vi "欧姆龙PLC通讯Main-TCP.vi"(9 "起始地址16":string="\u0000\u001e\u0000", 10 "数据":dbl[](array[numeric]), 11 "欧姆龙PLC Action":T1) -> (0 "接收数据":string, 1 "读取高度值":i16, 2 "触发信号":bool[](array[boolean]), 3 "PLC连线成功":bool)   [LabVIEW 2014]
uses:
  Controls/MsgAction.ctl
panel:
  out "数组 2":i16[](array[numeric])
  out "数组":i16[](array[numeric])
  out "布尔 2":bool
  out "无符号字节数组 2":u8[](array[numeric])
  out "子字符串 2":string
  out "错误输出 2":errorcluster caption="错误输出"
  in  "接收数据 参考":string="FINS\u0000\u0000\u0000\u001c\u0000\u0000\u0000\u0002\u0000\u0000\u0000\u0000€\u0000\u0002\u0000!\u0000\u0000À\u0000\u0000\u0001\u0002²\u0000\u001e\u0000\u0000\u0001\u0000\u0005"
  out "连接的字符串":string
  out "无符号字节数组":u8[](array[numeric])
  out "子字符串":string
  out "数据长度":string
  out "字符串":string
  out "布尔":bool
  out "错误输出":errorcluster
  out "打开TCP连接成功 2":bool
  out "打开TCP连接成功":bool
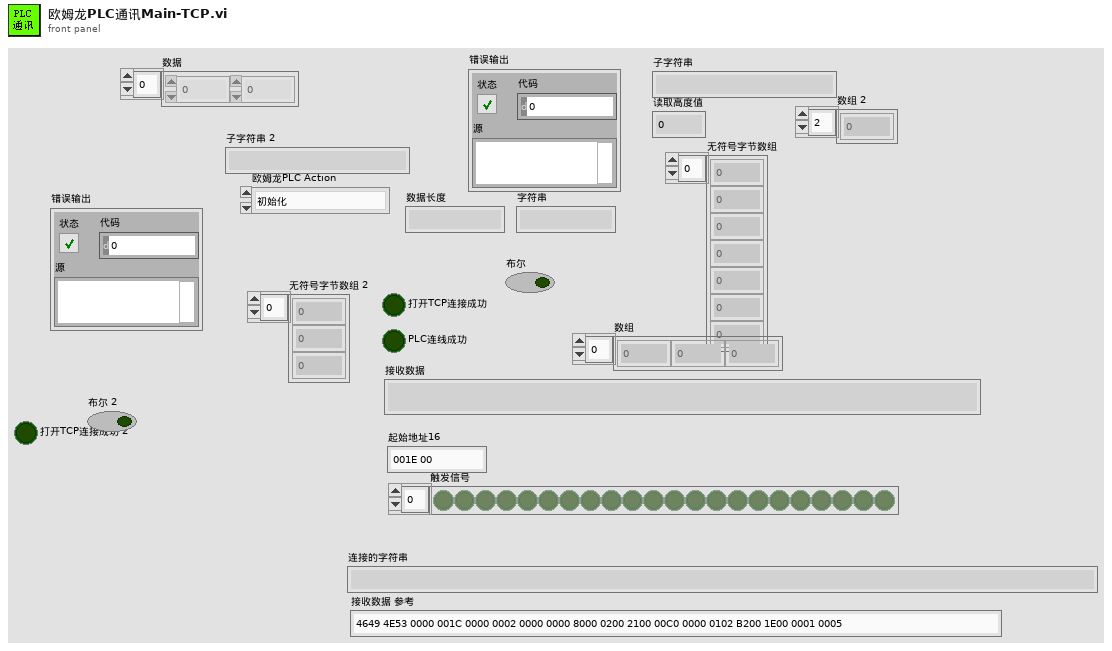
[diagram p1: front panel]
types:
  T1 = typedef "欧姆龙PLC Action.ctl" = enum16{"初始化", "重新初始化", "读触发信息", "读共面度", "写数据", "获取信息"}
  T2 = typedef "MsgAction.ctl" = enum16{"初始化", "添加消息", "区分结果添加消息", "清空消息", "获取消息"}
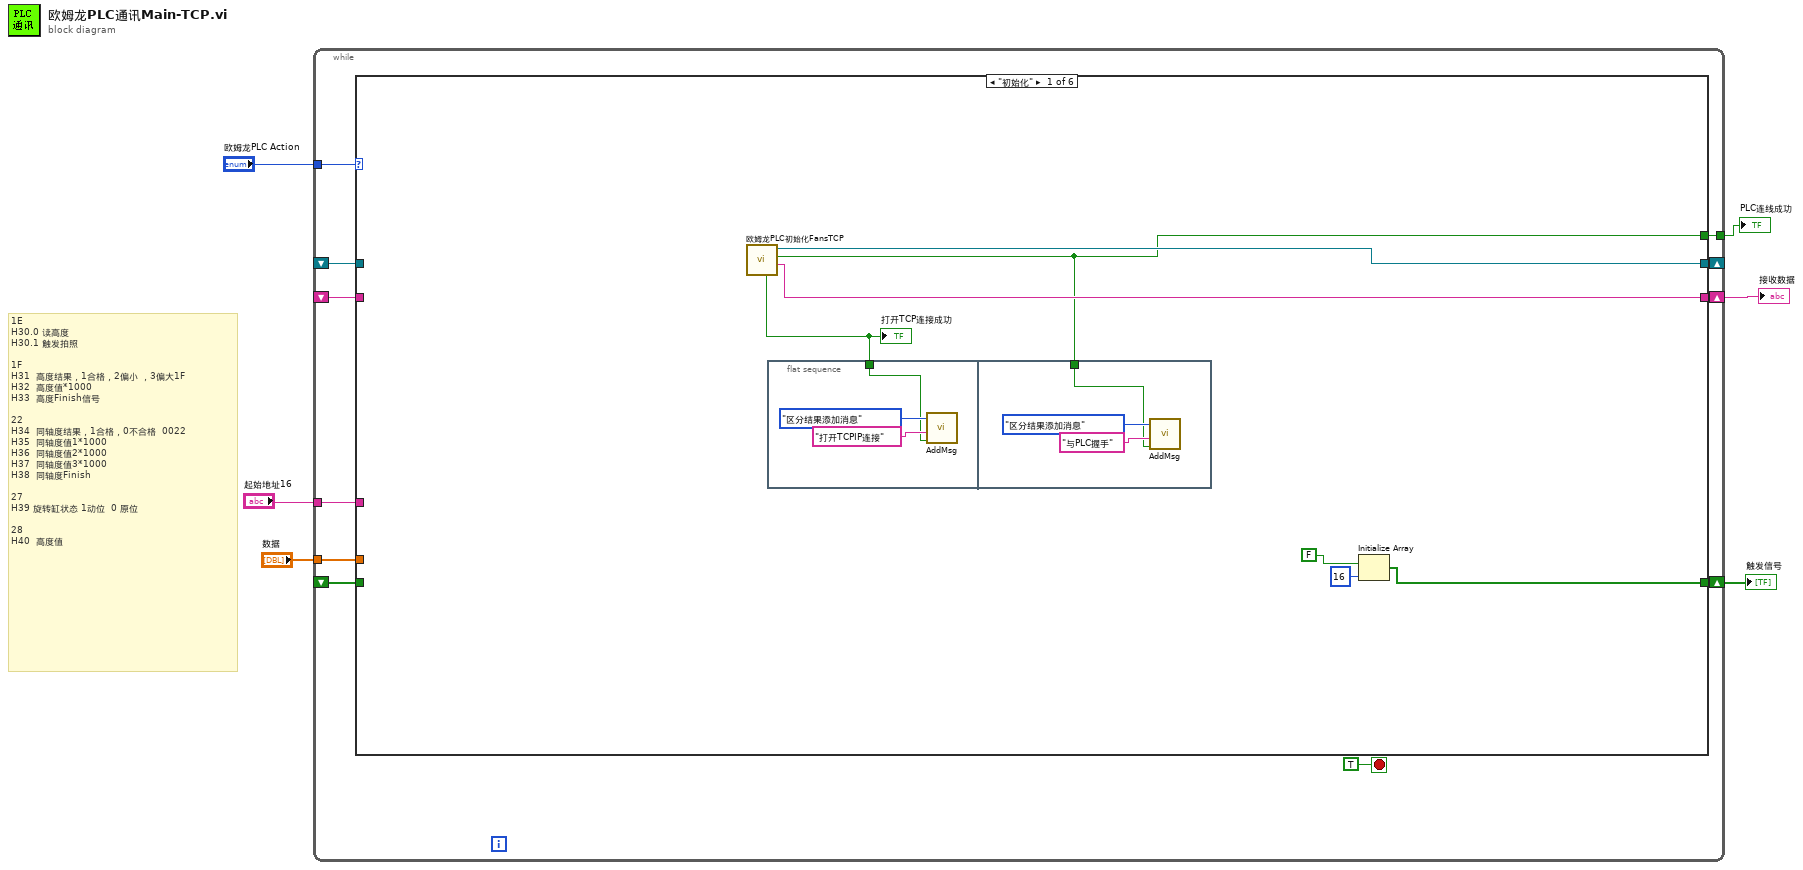
[diagram p0: block diagram]
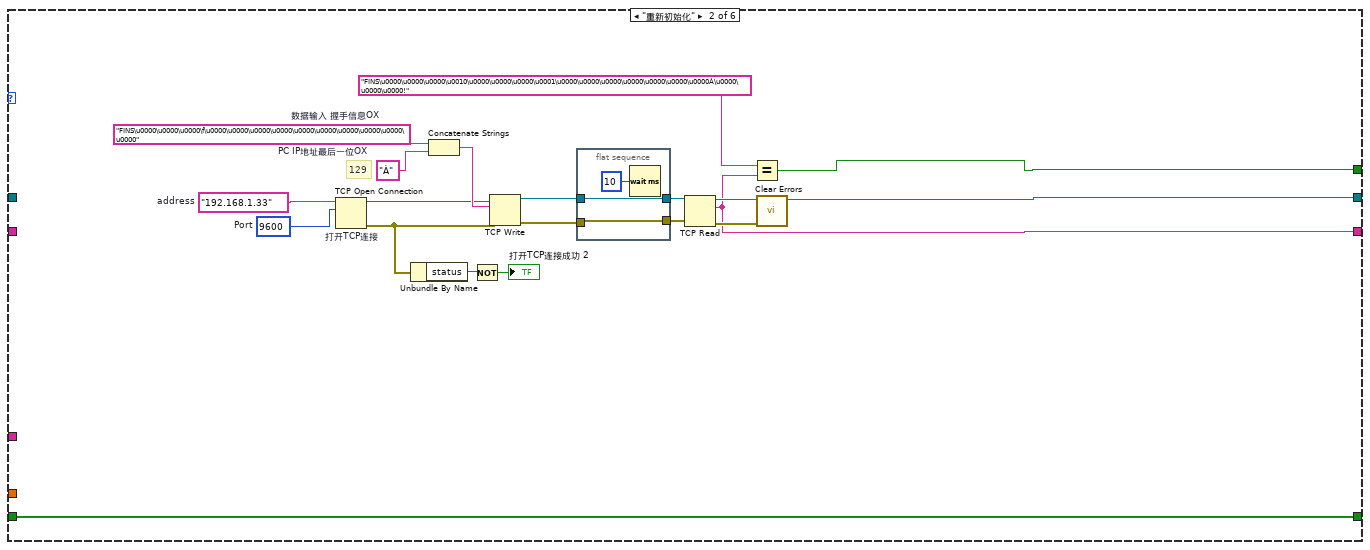
[diagram p2: hidden frame]
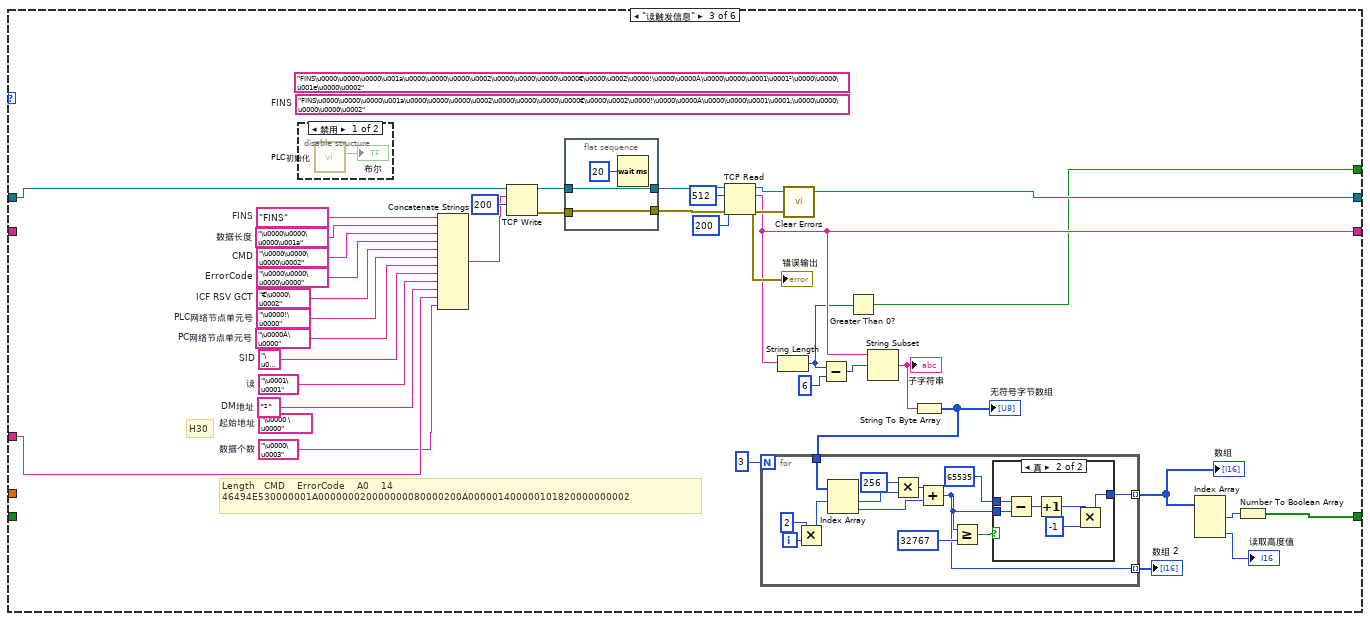
[diagram p3: hidden frame]
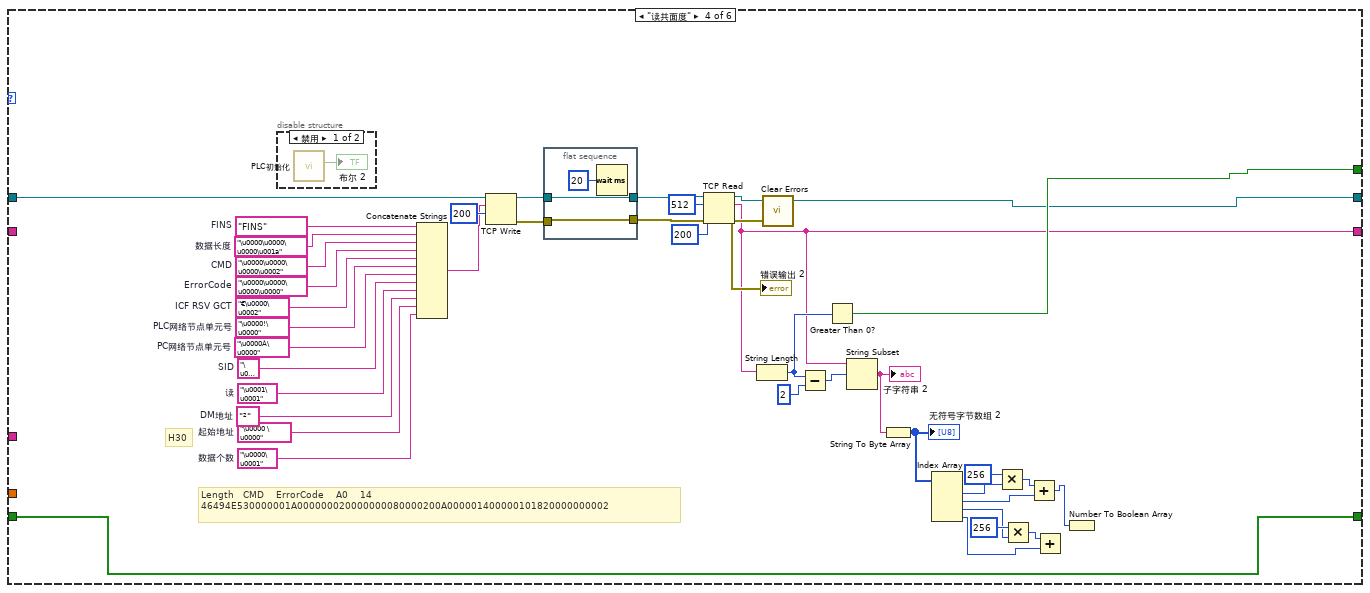
[diagram p6: hidden frame]
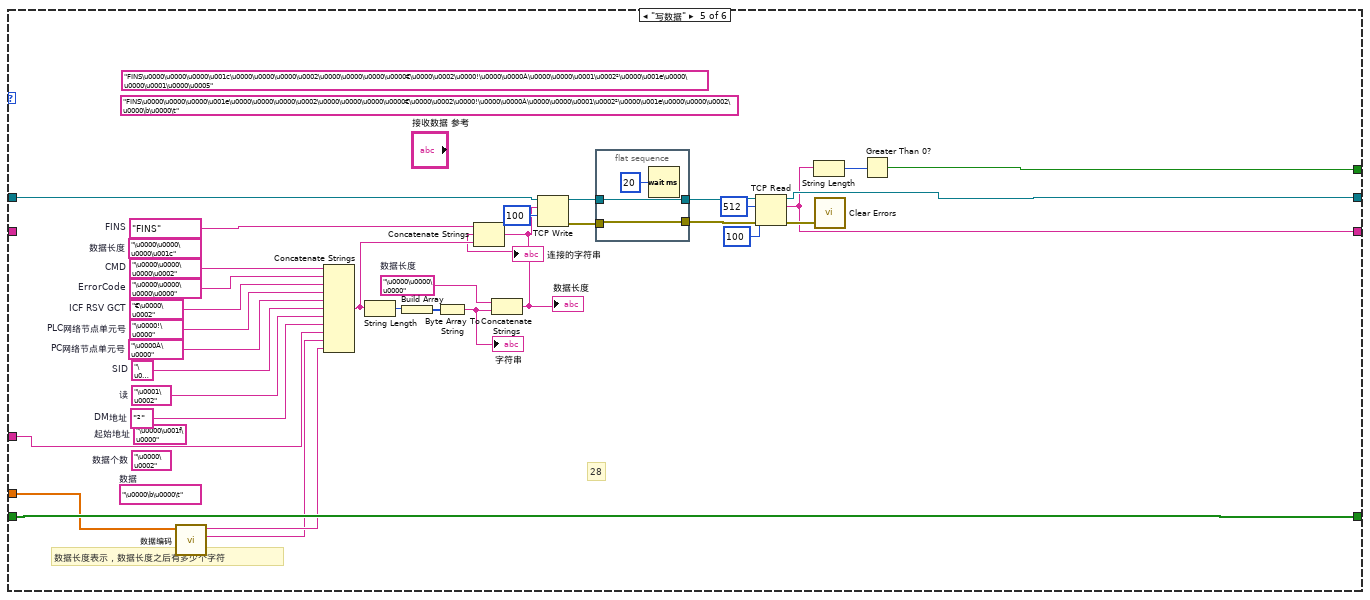
[diagram p8: hidden frame]
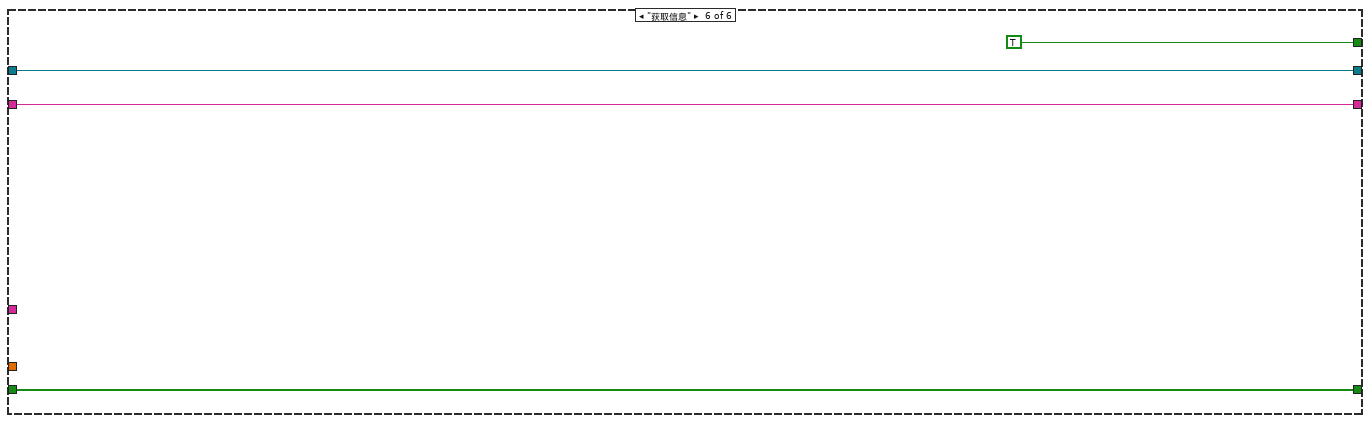
[diagram p9: hidden frame]
diagram:
  # "1E\nH30.0 读高度\nH30.1 触发拍照\n\n1F\nH31  高度结果，1合格，2偏小 ，3偏大1F\nH32  高度值*1000\nH33  高度Finish信号\n\n22\nH34  同轴度结果，1合格，0不合格  0022\nH35  同轴度值1*1000\nH36  同轴度值2*1000\nH37  同轴度值3*1000\nH38  同轴度Finish\n\n27\nH39 旋转缸状态 1动位  0 原位\n\n28\nH40  高度值"
  n1 = while {
    tunnel: "欧姆龙PLC Action" -> [w16]
    shift-right: [w15] -> _
    shift-left: _ -> [w14]
    shift-right: [w13] -> w5
    shift-left: _ -> [w12]
    tunnel: [w11] -> w4
    shift-right: [w10] -> w3
    shift-left: _ -> [w9]
    tunnel: "起始地址16" -> [w8]
    tunnel: "数据" -> [w7]
    stop <- TRUE ("停止") stop-if-true
    n2 = case shown="\"初始化\"" w16 {
      tunnel: [w24 w34 w74 w117 w174 w197] -> w15
      tunnel: w14 -> [_ _ w61 w119 w162 w197]
      tunnel: [w23 w33 w68 w116 w165 w196] -> w13
      tunnel: w12 -> [_ _ _ _ _ w196]
      tunnel: [w18 w32 w62 w118 w163 TRUE ("布尔")] -> w11
      tunnel: [w20 w31 w64 w114 w166 w194] -> w10
      tunnel: w9 -> [_ w31 _ w114 w166 w194]
      tunnel: w8 -> [_ _ w60 _ w161 _]
      tunnel: w7 -> [_ _ _ _ w158 _]
      frame "初始化" {
        n3 = call "欧姆龙PLC初始化FansTCP.vi"() -> ("data out"=w23:string, "布尔"=w18:bool, "TCP网络连接输出"=w24:refnum<k5>, "打开TCP连接成功"=w19:bool)  [unwired: 8 in]
        "打开TCP连接成功" <- w19
        n4 = flat-sequence {
          tunnel: w19 -> [w25]
          tunnel: w18 -> [w28]
          frame #0 {
            n5 = call "AddMsg.vi"("Result"=w25, "添加消息"="打开TCPIP连接" ("消息显示"), "消息Action"=MsgAction."区分结果添加消息") -> ()  [unwired: 1 in, 1 out]
          }
          frame #1 {
            n6 = call "AddMsg.vi"("Result"=w28, "添加消息"="与PLC握手" ("消息显示"), "消息Action"=MsgAction."区分结果添加消息") -> ()  [unwired: 1 in, 1 out]
          }
        }
        n7 = Initialize Array(FALSE, 16 ("维数大小")) -> (w20:bool[])
      }
      frame "重新初始化" {
        w46 = "À"  # PC IP地址最后一位OX
        w47 = "FINS\u0000\u0000\u0000\f\u0000\u0000\u0000\u0000\u0000\u0000\u0000\u0000\u0000\u0000"  # 数据输入 握手信息OX
        w48 = 9600  # Port
        w49 = "192.168.1.33"  # address
        # "129"
        n8 = TCP Open Connection "打开TCP连接"(address=w49, remote port or service name=w48) -> (connection ID=w42:refnum<k5>, error out=w41:errorcluster)  [unwired: 3 in]
        n9 = Unbundle By Name(w41) -> ("status"=w43:bool)
        n10 = Concatenate Strings(w47, w46) -> (w45:string)
        n11 = Not(x=w43) -> (.not. x?=→"打开TCP连接成功 2":bool)
        n12 = TCP Write(connection ID=w42, data in=w45, error in (no error)=w41) -> (connection ID out=w37:refnum<k5>, error out=w39:errorcluster)  [unwired: 1 in, 1 out]
        n13 = flat-sequence {
          tunnel: w39 -> [w52]
          tunnel: [w52] -> w38
          tunnel: w37 -> [w50]
          tunnel: [w50] -> w36
          frame #0 {
            n14 = Wait (ms)(milliseconds to wait=u32 10 ("等待时间（毫秒）")) -> ()  [unwired: 1 out]
          }
        }
        n15 = TCP Read(connection ID=w36, error in (no error)=w38) -> (connection ID out=w34:refnum<k5>, data out=w33:string, error out=w40:errorcluster)  [unwired: 3 in]
        n16 = Equal?(x="FINS\u0000\u0000\u0000\u0010\u0000\u0000\u0000\u0001\u0000\u0000\u0000\u0000\u0000\u0000\u0000À\u0000\u0000\u0000!", y=w33) -> (x = y?=w32:bool)
        n17 = call <vilib>:"Clear Errors.vi"("error in (no error)"=w40) -> ()  [unwired: 5 in, 2 out]
      }
      frame "读触发信息" {
        (unwired) "FINS\u0000\u0000\u0000\u001a\u0000\u0000\u0000\u0002\u0000\u0000\u0000\u0000€\u0000\u0002\u0000!\u0000\u0000À\u0000\u0000\u0001\u0001²\u0000\u0000\u001e\u0000\u0002" ("接收数据 2")
        (unwired) "FINS\u0000\u0000\u0000\u001a\u0000\u0000\u0000\u0002\u0000\u0000\u0000\u0000€\u0000\u0002\u0000!\u0000\u0000À\u0000\u0000\u0001\u0001‚\u0000\u0000\u0000\u0000\u0002"  # FINS
        w59 = "\u0000\u0003"  # 数据个数
        (unwired) "\u0000 \u0000"  # 起始地址
        w79 = "²"  # DM地址
        w80 = "\u0001\u0001"  # 读
        w81 = "\u0000"  # SID
        w82 = "\u0000À\u0000"  # PC网络节点单元号
        w83 = "\u0000!\u0000"  # PLC网络节点单元号
        w84 = "€\u0000\u0002"  # ICF RSV GCT
        w85 = "\u0000\u0000\u0000\u0000"  # ErrorCode
        w86 = "\u0000\u0000\u0000\u0002"  # CMD
        w87 = "\u0000\u0000\u0000\u001a"  # 数据长度
        w88 = "FINS"  # FINS
        # "H30"
        # "Length   CMD    ErrorCode    A0    14\n46494E530000001A000000020000000080000200A000001400000101820000000002"
        n18 = disable-structure shown="禁用" {
          frame Disabled {
            n19 = call "PLC初始化.vi"() -> ("布尔"=→"布尔":bool)  [unwired: 8 in, 3 out]
          }
          frame Enabled {
          }
        }
        n20 = Concatenate Strings(w88, w87, w86, w85, w84, w83, w82, w81, w80, w79, w60, w59) -> (w69:string)
        n21 = TCP Write ("写入TCP数据")(connection ID=w61, data in=w69, 9:200 ("超时毫秒(25000)")) -> (connection ID out=w76:refnum<k5>, error out=w75:errorcluster)  [unwired: 1 in, 1 out]
        n22 = flat-sequence {
          tunnel: w75 -> [w112]
          tunnel: [w112] -> w78
          tunnel: w76 -> [w110]
          tunnel: [w110] -> w77
          frame #0 {
            n23 = Wait (ms)(milliseconds to wait=u32 20 ("等待时间（毫秒）")) -> ()  [unwired: 1 out]
          }
        }
        n24 = TCP Read(connection ID=w77, bytes to read=512 ("读取的字节"), error in (no error)=w78, 9:200 ("超时毫秒(25000)")) -> (connection ID out=w74:refnum<k5>, data out=w68:string, error out=w73:errorcluster)  [unwired: 1 in]
        "错误输出" <- w73
        n25 = String Length(string=w68) -> (length=w63:i32)
        n26 = call <vilib>:"Clear Errors.vi"("error in (no error)"=w73) -> ()  [unwired: 5 in, 2 out]
        n27 = Subtract(x=w63, y=6) -> (x-y=w66:i32)
        n28 = Greater Than 0?(x=w63) -> (x > 0?=w62:bool)
        n29 = String Subset(string=w68, offset (0)=w66) -> (substring=w65:string)  [unwired: 1 in]
        "子字符串" <- w65
        n30 = String To Byte Array(string=w65) -> (unsigned byte array=w55:u8[])
        "无符号字节数组" <- w55
        n31 = for {
          N: 3 -> [_]
          tunnel: w55 -> [w101]
          tunnel: [w90] -> w54 mode=indexing
          tunnel: [w89] -> w53 mode=indexing
          i -> [w96]
          n32 = Multiply(x=2, y=w96) -> (x*y=w94:i32)
          n33 = Index Array(array=w101, index #1=w94) -> (element #1=w100:u8, element #2=w98:u8)  [unwired: 1 in]
          n34 = Multiply(x=u16 256, y=w100) -> (x*y=w99:u16)
          n35 = Add(x=w99, y=w98) -> (x+y=w89:u16)
          n36 = Greater Or Equal?(x=w89, y=i16 32767) -> (x >= y?=w92:bool)
          n37 = case shown="真" w92 {
            tunnel: u16 65535 -> [_ w108]
            tunnel: w89 -> [w102 w107]
            tunnel: [w102 w103] -> w90
            frame False {
            }
            frame True {
              n38 = Subtract(x=w108, y=w107) -> (x-y=w106:u16)
              n39 = Increment(x=w106) -> (x+1=w105:u16)
              n40 = Multiply(x=w105, y=i16 -1) -> (x*y=w103:u16)
            }
          }
        }
        "数组" <- w54
        "数组 2" <- w53
        n41 = Index Array(array=w54) -> (element #1=w58:u16, element #3=→"读取高度值":u16)  [unwired: 3 in, 1 out]
        n42 = Number To Boolean Array(number=w58) -> (Boolean array=w64:bool[])
      }
      frame "读共面度" {
        w142 = "\u0000\u0001"  # 数据个数
        w113 = "\u0000 \u0000"  # 起始地址
        w143 = "²"  # DM地址
        w144 = "\u0001\u0001"  # 读
        w145 = "\u0000"  # SID
        w146 = "\u0000À\u0000"  # PC网络节点单元号
        w147 = "\u0000!\u0000"  # PLC网络节点单元号
        w148 = "€\u0000\u0002"  # ICF RSV GCT
        w149 = "\u0000\u0000\u0000\u0000"  # ErrorCode
        w150 = "\u0000\u0000\u0000\u0002"  # CMD
        w151 = "\u0000\u0000\u0000\u001a"  # 数据长度
        w152 = "FINS"  # FINS
        # "H30"
        # "Length   CMD    ErrorCode    A0    14\n46494E530000001A000000020000000080000200A000001400000101820000000002"
        n43 = disable-structure shown="禁用" {
          frame Disabled {
            n44 = call "PLC初始化.vi"() -> ("布尔"=→"布尔 2":bool)  [unwired: 8 in, 3 out]
          }
          frame Enabled {
          }
        }
        n45 = Concatenate Strings(w152, w151, w150, w149, w148, w147, w146, w145, w144, w143, w113, w142) -> (w133:string)
        n46 = TCP Write ("写入TCP数据")(connection ID=w119, data in=w133, 9:200 ("超时毫秒(25000)")) -> (connection ID out=w139:refnum<k5>, error out=w138:errorcluster)  [unwired: 1 in, 1 out]
        n47 = flat-sequence {
          tunnel: w138 -> [w156]
          tunnel: [w156] -> w141
          tunnel: w139 -> [w154]
          tunnel: [w154] -> w140
          frame #0 {
            n48 = Wait (ms)(milliseconds to wait=u32 20 ("等待时间（毫秒）")) -> ()  [unwired: 1 out]
          }
        }
        n49 = TCP Read(connection ID=w140, bytes to read=512 ("读取的字节"), error in (no error)=w141, 9:200 ("超时毫秒(25000)")) -> (connection ID out=w117:refnum<k5>, data out=w116:string, error out=w137:errorcluster)  [unwired: 1 in]
        "错误输出 2" <- w137
        n50 = String Length(string=w116) -> (length=w124:i32)
        n51 = call <vilib>:"Clear Errors.vi"("error in (no error)"=w137) -> ()  [unwired: 5 in, 2 out]
        n52 = Subtract(x=w124, y=2) -> (x-y=w131:i32)
        n53 = Greater Than 0?(x=w124) -> (x > 0?=w118:bool)
        n54 = String Subset(string=w116, offset (0)=w131) -> (substring=w130:string)  [unwired: 1 in]
        "子字符串 2" <- w130
        n55 = String To Byte Array(string=w130) -> (unsigned byte array=w129:u8[])
        "无符号字节数组 2" <- w129
        n56 = Index Array(array=w129) -> (element #1=w128:u8, element #2=w126:u8, element #3=w121:u8, element #4=w120:u8)  [unwired: 4 in]
        n57 = Multiply(x=u16 256, y=w128) -> (x*y=w127:u16)
        n58 = Multiply(x=u16 256, y=w121) -> (x*y=w122:u16)
        n59 = Add(x=w127, y=w126) -> (x+y=w115:u16)
        n60 = Add(x=w122, y=w120) -> ()  [unwired: 1 out]
        n61 = Number To Boolean Array(number=w115) -> ()  [unwired: 1 out]
      }
      frame "写数据" {
        (unwired) "FINS\u0000\u0000\u0000\u001e\u0000\u0000\u0000\u0002\u0000\u0000\u0000\u0000€\u0000\u0002\u0000!\u0000\u0000À\u0000\u0000\u0001\u0002²\u0000\u001e\u0000\u0000\u0002\u0000\b\u0000\t" ("连接的字符串")
        (unwired) "\u0000\b\u0000\t"  # 数据
        w172 = "\u0000\u0000\u0000"  # 数据长度
        (unwired) "FINS\u0000\u0000\u0000\u001c\u0000\u0000\u0000\u0002\u0000\u0000\u0000\u0000€\u0000\u0002\u0000!\u0000\u0000À\u0000\u0000\u0001\u0002²\u0000\u001e\u0000\u0000\u0001\u0000\u0005" ("接收数据 3")
        (unwired) "\u0000\u0002"  # 数据个数
        (unwired) "\u0000\u001f\u0000"  # 起始地址
        w183 = "²"  # DM地址
        w184 = "\u0001\u0002"  # 读
        w185 = "\u0000"  # SID
        w186 = "\u0000À\u0000"  # PC网络节点单元号
        w187 = "\u0000!\u0000"  # PLC网络节点单元号
        w188 = "€\u0000\u0002"  # ICF RSV GCT
        w189 = "\u0000\u0000\u0000\u0000"  # ErrorCode
        w190 = "\u0000\u0000\u0000\u0002"  # CMD
        (unwired) "\u0000\u0000\u0000\u001c"  # 数据长度
        w173 = "FINS"  # FINS
        # "数据长度表示，数据长度之后有多少个字符"
        # "28"
        n62 = call "数据编码.vi"("数据"=w158) -> ("数据个数"=w157:string, "字符串"=w159:string)  [unwired: 9 in]
        n63 = Concatenate Strings(w190, w189, w188, w187, w186, w185, w184, w183, w161, w157, w159) -> (w171:string)
        n64 = String Length(string=w171) -> (length=w169:i32)
        n65 = Build Array(w169) -> (w168:i32[])
        n66 = Byte Array To String(unsigned byte array=w168) -> (string=w167:string)
        "字符串" <- w167
        n67 = Concatenate Strings(w172, w167) -> (w170:string)
        "数据长度" <- w170
        n68 = Concatenate Strings(w173, w170, w171) -> (w160:string)
        "连接的字符串" <- w160
        n69 = TCP Write ("写入TCP数据")(connection ID=w162, data in=w160, 9:100 ("超时毫秒(25000)")) -> (connection ID out=w180:refnum<k5>, error out=w179:errorcluster)  [unwired: 1 in, 1 out]
        n70 = flat-sequence {
          tunnel: w179 -> [w193]
          tunnel: [w193] -> w182
          tunnel: w180 -> [w191]
          tunnel: [w191] -> w181
          frame #0 {
            n71 = Wait (ms)(milliseconds to wait=u32 20 ("等待时间（毫秒）")) -> ()  [unwired: 1 out]
          }
        }
        n72 = TCP Read(connection ID=w181, bytes to read=512 ("读取的字节"), error in (no error)=w182, 9:100 ("超时毫秒(25000)")) -> (connection ID out=w174:refnum<k5>, data out=w165:string, error out=w178:errorcluster)  [unwired: 1 in]
        n73 = String Length(string=w165) -> (length=w164:i32)
        n74 = call <vilib>:"Clear Errors.vi"("error in (no error)"=w178) -> ()  [unwired: 5 in, 2 out]
        n75 = Greater Than 0?(x=w164) -> (x > 0?=w163:bool)
      }
      frame "获取信息" {
      }
    }
  }
  "接收数据" <- w5
  "PLC连线成功" <- w4
  "触发信号" <- w3
